vi "CheckOnIdle.vi"(7 "OverwriteClass? (F)":bool, 8 "error in (no error)":errorcluster, 9 "Timeout (s)":dbl=5.0 min=0.0 max=5.0, 10 "ChangeOccured? (F)":bool, 11 "SpecAnPlugins.lvlib In":refnum<class "SpecAnBase.lvclass">) -> (0 "Error Out":errorcluster, 2 "Write?":bool, 3 "SpecAnPlugins.lvlib In 2":refnum<class "SpecAnBase.lvclass">)   [LabVIEW 2018, in "SpecAnModule.lvlib"]
doc: "This VI checks to make sure the acquisition loop is in the idle state before we set the write boolean to True. This boolean can be used in conjunction with the Class Action Node in order to overwrite the properties of the class plugin. The overwrite class boolean must be set to true otherwise the write boolean will return a flase. The VI will only check if the VI is in the idle state for the amount of time specified in the Timeout countrol and throw an error if this time is exceeded. The default value for this control is five seconds."
uses:
  SpecAnModule.lvlib
  SpecAnPlugins/SpecAnBaseClass/SpecAnBase.lvclass
  <vilib>/Utility/error.llb/Error Cluster From Error Code.vi
  <vilib>/ErrorRing/Error Ring.xnode
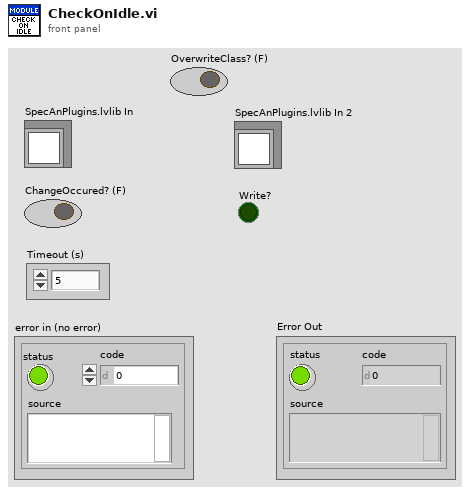
[diagram p1: front panel]
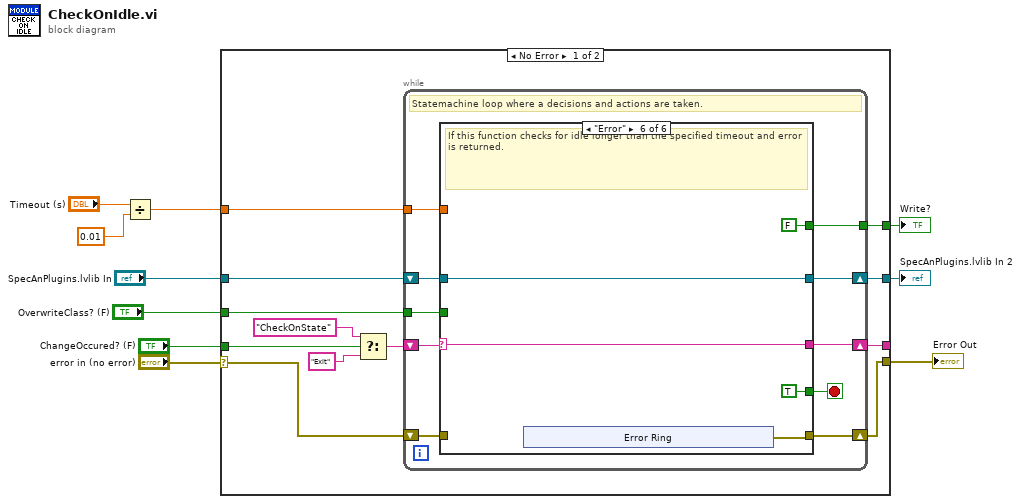
[diagram p0: block diagram]
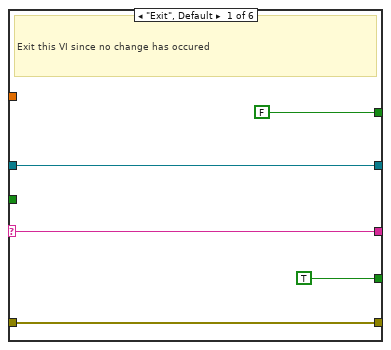
[diagram p2: hidden frame]
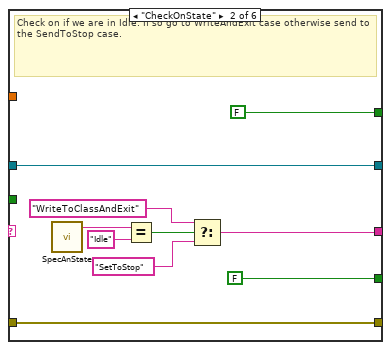
[diagram p3: hidden frame]
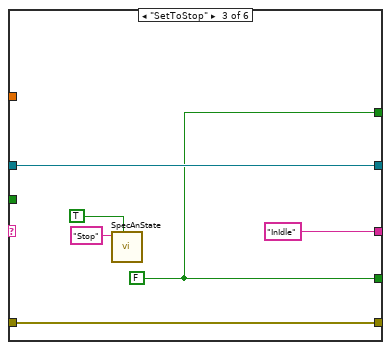
[diagram p4: hidden frame]
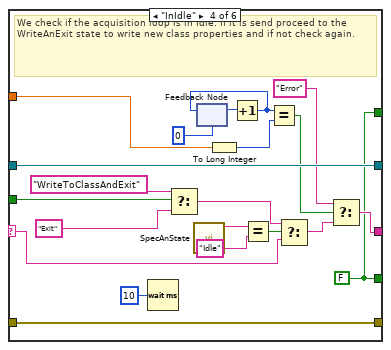
[diagram p5: hidden frame]
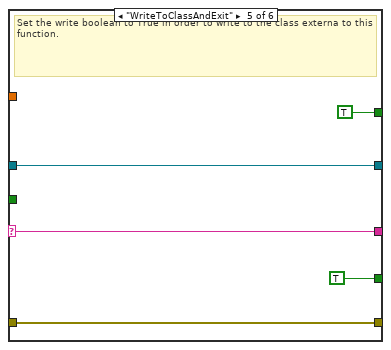
[diagram p6: hidden frame]
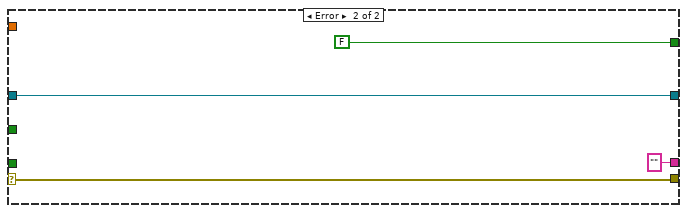
[diagram p7: hidden frame]
diagram:
  n1 = Divide(x="Timeout (s)", y=0.01) -> (x/y=w3:dbl)
  n2 = case shown="No Error" "error in (no error)" {
    selector: "error in (no error)" -> [w19 w93]
    tunnel: "ChangeOccured? (F)" -> [w18 _]
    tunnel: "SpecAnPlugins.lvlib In" -> [w17 w92]
    tunnel: [w16 w93] -> w10
    tunnel: "OverwriteClass? (F)" -> [w15 _]
    tunnel: w3 -> [w14 _]
    tunnel: [w13 w92] -> w2
    tunnel: [w12 FALSE ("Set? (f)")] -> w1
    tunnel: [w11 "" ("y")] -> _
    frame No Error {
      n3 = Select(t="CheckOnState" ("y"), s=w18, f="Exit" ("y")) -> (s? t:f=w22:string)
      n4 = while {
        shift-right: [w27] -> w11
        shift-left: w22 -> [w32]
        shift-right: [w29] -> w13
        shift-left: w17 -> [w30]
        shift-right: [w28] -> w16
        shift-left: w19 -> [w31]
        tunnel: w15 -> [w25]
        tunnel: w14 -> [w24]
        tunnel: [w23] -> w12
        stop <- w26 stop-if-true
        # "Statemachine loop where a decisions and actions are taken."
        n5 = case shown="\"Error\"" w32 {
          selector: w32 -> [w36 _ _ w71 w77 w83]
          tunnel: w31 -> [w37 w45 w51 w70 w79 _]
          tunnel: w30 -> [w35 w44 w50 w69 w76 w82]
          tunnel: [w37 w45 w51 w70 w79 w81] -> w28
          tunnel: [w35 w44 w50 w69 w76 w82] -> w29
          tunnel: [w36 w42 "InIdle" ("y") w60 w77 w83] -> w27
          tunnel: [TRUE FALSE w48 w54 TRUE TRUE] -> w26
          tunnel: w25 -> [_ _ _ w63 _ _]
          tunnel: w24 -> [_ _ _ w55 _ _]
          tunnel: [FALSE ("Set? (f)") FALSE ("Set? (f)") w48 w54 TRUE ("Set? (f)") FALSE ("Set? (f)")] -> w23
          frame "Exit", Default {
            # "Exit this VI since no change has occured"
          }
          frame "CheckOnState" {
            # "Check on if we are in Idle. If so go to WriteAndExit case otherwise send to the SendToStop case."
            n6 = call "SpecAnState.vi"() -> ("State Out"=w47:string)  [unwired: 11 in]
            n7 = Equal?(x=w47, y="Idle") -> (x = y?=w43:bool)
            n8 = Select(t="WriteToClassAndExit" ("y"), s=w43, f="SetToStop" ("y")) -> (s? t:f=w42:string)
          }
          frame "SetToStop" {
            w48 = FALSE
            n9 = call "SpecAnState.vi"("Set Boolean"=TRUE, "State In"="Stop") -> ()  [unwired: 9 in, 1 out]
          }
          frame "InIdle" {
            w54 = FALSE
            # "We check if the acquisition loop is in Idle. If it is send proceed to the WriteAnExit state to write new class properties and if not check again."
            n10 = Wait (ms)(milliseconds to wait=u32 10) -> ()  [unwired: 1 out]
            n11 = Select(t="WriteToClassAndExit" ("State In"), s=w63, f="Exit" ("State In")) -> (s? t:f=w64:string)
            n12 = call "SpecAnState.vi"() -> ("State Out"=w74:string)  [unwired: 11 in]
            n13 = feedback #1(0) -> (w67:i32)
            n14 = To Long Integer(number=w55) -> (32bit integer=w56:i32)
            n15 = Increment(x=w67) -> (x+1=w66:i32)
            n16 = feedback-in #1(w66) -> ()
            n17 = Equal?(x=w74, y="Idle" ("State In")) -> (x = y?=w72:bool)
            n18 = Equal?(x=w66, y=w56) -> (x = y?=w59:bool)
            n19 = Select(t=w64, s=w72, f=w71) -> (s? t:f=w61:string)
            n20 = Select(t="Error" ("State In"), s=w59, f=w61) -> (s? t:f=w60:string)
          }
          frame "WriteToClassAndExit" {
            # "Set the write boolean to True in order to write to the class externa to this function."
          }
          frame "Error" {
            # "If this function checks for idle longer than the specified timeout and error is returned."
            n21 = xnode "Error Ring"() -> ("error out"=w81:errorcluster)
          }
        }
      }
    }
    frame Error {
    }
  }
  "Error Out" <- w10
  "SpecAnPlugins.lvlib In 2" <- w2
  "Write?" <- w1
